vi "MGI Set String Scrollbar.vi"(10 "Error In":errorcluster, 11 "String Reference":refnum<vi>) -> (2 "Error Out":errorcluster, 3 "String Reference(dup)":refnum<vi>)   [LabVIEW 2016]
doc: "Show or hide the specified string control's vertical scrollbar based on the contents of the string control. This VI will also set the scrollbar position as necessary to ensure that some of the string is displayed.\nIf the string control does not enable wrapping, then the horizontal scrollbar may also be shown or hidden based on the length of the longest line in the string.\n\nAuthored by Shawn Walpole\nsupport@mooregoodideas.com\nwww.mooregoodideas.com\n\nCopyright (c) 2010, Moore Good Ideas, Inc.\n\nAll rights reserved.\n\nRedistribution and use in source and binary forms, with or without modification, are permitted provided that the following conditions are met:\n\n * Redistributions of source code must retain the above copyright notice, this list of conditions and the following disclaimer.\n * Redistributions in binary form must reproduce the above copyright notice, this list of conditions and the following disclaimer in the documentation and/or other materials provided with the distribution.\n * Neither the name of Moore Good Ideas, Inc. nor the names of its contributors may be used to endorse or promote products derived from this software without specific prior written permission.\n\nTHIS SOFTWARE IS PROVIDED BY THE COPYRIGHT HOLDERS AND CONTRIBUTORS \"AS IS\" AND ANY EXPRESS OR IMPLIED WARRANTIES, INCLUDING, BUT NOT LIMITED TO, THE IMPLIED WARRANTIES OF MERCHANTABILITY AND FITNESS FOR A PARTICULAR PURPOSE ARE DISCLAIMED. IN NO EVENT SHALL THE COPYRIGHT OWNER OR CONTRIBUTORS BE LIABLE FOR ANY DIRECT, INDIRECT, INCIDENTAL, SPECIAL, EXEMPLARY, OR CONSEQUENTIAL DAMAGES (INCLUDING, BUT NOT LIMITED TO, PROCUREMENT OF SUBSTITUTE GOODS OR SERVICES; LOSS OF USE, DATA, OR PROFITS; OR BUSINESS INTERRUPTION) HOWEVER CAUSED AND ON ANY THEORY OF LIABILITY, WHETHER IN CONTRACT, STRICT LIABILITY, OR TORT (INCLUDING NEGLIGENCE OR OTHERWISE) ARISING IN ANY WAY OUT OF THE USE OF THIS SOFTWARE, EVEN IF ADVISED OF THE POSSIBILITY OF SUCH DAMAGE."
panel:
  in  "[user-specified font]":T1
  out "result":cluster{"Left":i32, "Top":i32}
  out "length":i32
  out "Byte offset (Vertical)":i32
  # "Debugging Controls:"
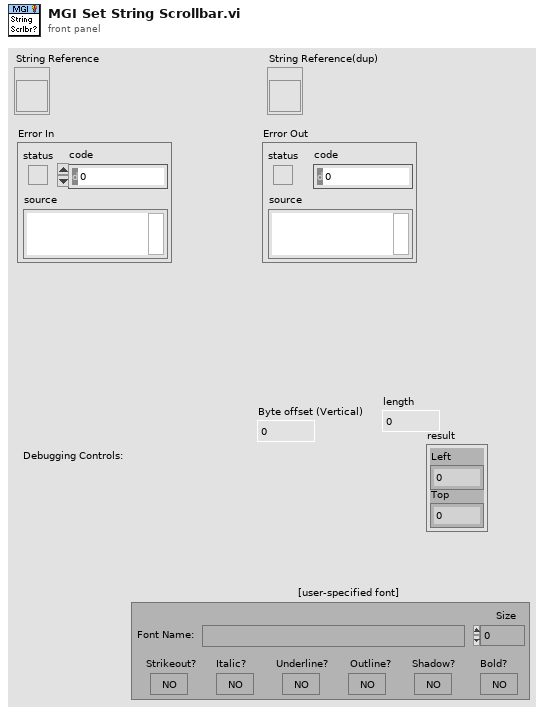
[diagram p1: front panel]
types:
  T1 = cluster{"Font Name:":string, "Size":i16, "Strikeout?":bool, "Italic?":bool, "Underline?":bool, "Outline?":bool, "Shadow?":bool, "Bold?":bool}
  T2 = typedef "LVBoundsTypeDef.ctl" = cluster{"Width":u32, "Height":u32}
  T3 = typedef "LVPositionTypeDef.ctl" = cluster{"Left":i32, "Top":i32}
  T4 = cluster{"horizontal":enum16{"left", "center", "right"}, "vertical":enum16{"top", "center", "bottom"}}
  T5 = enum16{"User-specified Font", "Application Font", "System Font", "Dialog Font"}
  T6 = typedef "LVFontTypeDef.ctl" = cluster{"Font Name":string, "Size":u16, "Bold":bool, "Italic":bool, "Underline":bool, "Strikeout":bool, "Color":u32}
  T7 = cluster{"left":i16, "top":i16, "right":i16, "bottom":i16}
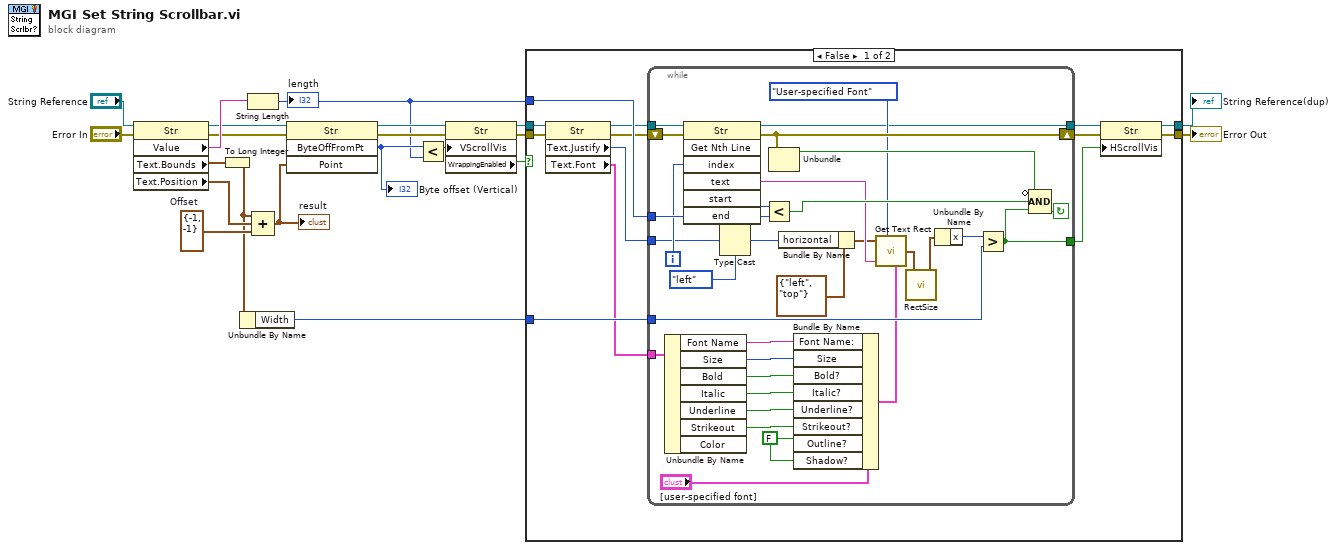
[diagram p0: block diagram]
diagram:
  w7 = cluster{"Left":i32, "Top":i32} {"Left"=-1, "Top"=-1}  # Offset
  n1 = property class="Str"(reference="String Reference", error in="Error In") -> (reference out=w9:refnum<vi>, error out=w10:errorcluster, "Value"=w20:string, "Text.Bounds"=w18:T2, "Text.Position"=w17:T3)
  n2 = To Long Integer(number=w18) -> (32bit integer=w5:cluster{"Width":i32, "Height":i32})
  n3 = Unbundle By Name(w5) -> ("Width"=w4:i32)
  n4 = String Length(string=w20) -> (length=w6:i32)
  "length" <- w6
  n5 = Compound Arithmetic op=ADD(w5, w17, w7) -> (w19:T3)
  "result" <- w19
  n6 = invoke class="Str" method="ByteOffFromPt"(reference=w9, error in=w10, "Point"=w19) -> (reference out=w15:refnum<vi>, error out=w16:errorcluster, "ByteOffFromPt"=w8:i32)  [unwired: 1 in, 1 out]
  "Byte offset (Vertical)" <- w8
  n7 = Less?(x=w8, y=w6) -> (x < y?=w14:bool)
  n8 = property class="Str"(reference=w15, error in=w16, "VScrollVis"=w14) -> (reference out=w13:refnum<vi>, error out=w12:errorcluster, "WrappingEnabled"=w11:bool)
  n9 = case shown="False" w11 {
    tunnel: w13 -> [w34 w68]
    tunnel: w12 -> [w33 w67]
    tunnel: w6 -> [w32 _]
    tunnel: w4 -> [w28 _]
    tunnel: [w24 w68] -> w3
    tunnel: [w23 w67] -> w2
    frame False {
      n10 = property class="Str"(reference=w34, error in=w33) -> (reference out=w31:refnum<vi>, error out=w30:errorcluster, "Text.Justify"=w29:enum16{"Left", "Center", "Right"}, "Text.Font"=w22:T6)
      n11 = while {
        tunnel: w32 -> [w65]
        tunnel: w31 -> [w64]
        shift-right: [w59] -> w26
        shift-left: w30 -> [w63]
        tunnel: w29 -> [w47]
        tunnel: [w51] -> w25
        tunnel: w28 -> [w50]
        tunnel: [w48] -> w27
        tunnel: w22 -> [w42]
        i -> [w49]
        stop <- w61 continue-if-true
        w35 = FALSE ("Outline?")
        n12 = Unbundle By Name(w42) -> ("Font Name"=w41:string, "Size"=w40:u16, "Bold"=w39:bool, "Italic"=w38:bool, "Underline"=w37:bool, "Strikeout"=w36:bool)  [unwired: 1 out]
        n13 = invoke class="Str" method="Get Nth Line"(reference=w64, error in=w63, "index"=w49) -> (reference out=w48:refnum<vi>, error out=w59:errorcluster, "text"=w58:string, "end"=w66:u32)  [unwired: 4 in, 3 out]
        n14 = Type Cast(type=enum16{"left", "center", "right"}."left" ("horizontal"), x=w47) -> (*(type *) &x=w46:enum16{"left", "center", "right"})
        n15 = Less?(x=w66, y=w65) -> (x < y?=w62:bool)
        n16 = Unbundle(w59) -> ("status"=w60:bool)  [unwired: 2 out]
        n17 = Bundle By Name(cluster=T4 {"horizontal"=enum."left", "vertical"=enum."top"} ("alignment(left, top)"), "horizontal"=w46) -> (w55:T4)
        n18 = Bundle By Name(cluster="[user-specified font]", "Font Name:"=w41, "Size"=w40, "Bold?"=w39, "Italic?"=w38, "Underline?"=w37, "Strikeout?"=w36, "Outline?"=w35, "Shadow?"=w35) -> (w44:T1)
        n19 = call <vilib>:"Get Text Rect.vi"("alignment(left, top)"=w55, "desired font(Application)"=T5."User-specified Font", "text"=w58, "[user-specified font]"=w44) -> ("rect"=w54:T7)  [unwired: 5 in]
        n20 = call <vilib>:"RectSize.vi"("rect"=w54) -> ("point"=w53:cluster{"x":i16, "y":i16})
        n21 = Unbundle By Name(w53) -> ("x"=w52:i16)
        n22 = Greater?(x=w52, y=w50) -> (0:w51:bool)
        n23 = Compound Arithmetic op=AND(invert w60, w62, w51) -> (w61:bool)
      }
      n24 = property class="Str"(reference=w27, error in=w26, "HScrollVis"=w25) -> (reference out=w24:refnum<vi>, error out=w23:errorcluster)
    }
    frame True {
    }
  }
  "String Reference(dup)" <- w3
  "Error Out" <- w2
